vi "Subvi trigger AO DO.vi"(9 "Ext trig enable":bool) -> ()   [LabVIEW 2017]
uses:
  <vilib>/Platform/TimedLoop/XDataNode/timing_clust.ctl
  <vilib>/Platform/TimedLoop/XDataNode/nitl_modes.ctl
  <vilib>/Platform/TimedLoop/XDataNode/wakeup.ctl
  <vilib>/rvi/Emulation/niFpgaSctlEmulationGetInTimedLoop.vi
  <vilib>/rvi/Emulation/niFpgaEmulationReportErrorSimple.vi
  <vilib>/rvi/Emulation/niFpgaGetClockAttributes.vi
  <vilib>/rvi/Emulation/niFpgaCriticalErrorInLSC.vi
  Detector/GV preline gate.vi
  GV trigger delay.vi
  <vilib>/Platform/TimedLoop/XDataNode/XDataNode.xnode
  <vilib>/Platform/TimedLoop/XDataNode/XDNodeRunTimeDep.lvlib
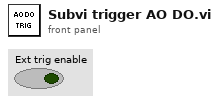
[diagram p1: front panel]
types:
  T1 = typedef "XDNodeRunTimeDep.lvlib/timing_clust.ctl" = cluster{"Expected End [f-1]":u64, "Actual End [f-1]":u64, "Finished Late? [f-1]":bool, "Expected End [i-1]":u64, "Actual End [i-1]":u64, "Finished Late? [i-1]":bool, "Expected Start [i]":u64, "Actual Start [i]":u64, "Expected Start [f]":u64, "Actual Start [f]":u64, "Source Name":string, "Structure Name":string, "Period":i64, "Deadline":i64, "Offset":i64, "Start":i64, "Priority":i32, "Timeout":i32, "Mode":T2, "Wakeup Reason":T3, "Error":errorcluster, "Source Type":string, "Secondary Source Type":string, "Global End Time":u64, "Global Start Time":u64, "Frame Duration":u64, "Iteration Duration":u64, "Assigned CPU":i32, "I/O Scan Engine Mode":u32}
  T2 = typedef "XDNodeRunTimeDep.lvlib/nitl_modes.ctl" = enum32{"No Change", "Process missed periods, maintain original phase", "Discard missed periods, maintain original phase", "Process missed periods, ignore original phase", "Discard missed periods, ignore original phase"}
  T3 = typedef "XDNodeRunTimeDep.lvlib/wakeup.ctl" = enum32{"Normal", "Aborted", "Asynchronous wakeup", "Timing source error", "Timed loop error", "Timeout"}
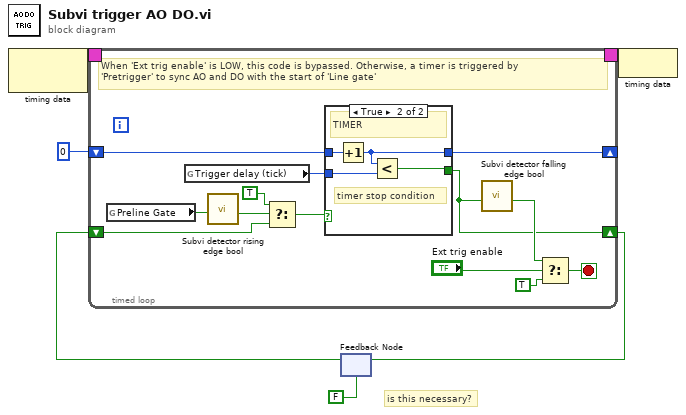
[diagram p0: block diagram]
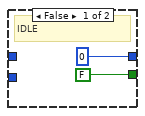
[diagram p2: hidden frame]
diagram:
  # "is this necessary?"
  n1 = node-c288() -> (w6:T1)  [unwired: 1 in]
  n2 = feedback #1(FALSE) -> (w2:bool)
  n3 = timed-loop {
    timing: w6 -> [_]
    timing-out: [_] -> w5
    shift-right: [w7] -> w1
    shift-left: w2 -> [w13]
    shift-right: [w16] -> _
    shift-left: u16 0 -> [w15]
    stop <- w11 stop-if-true
    # "When 'Ext trig enable' is LOW, this code is bypassed. Otherwise, a timer is triggered by\n'Pretrigger' to sync AO and DO with the start of 'Line gate'"
    n4 = global read "GV preline gate.vi" "Preline Gate"() -> (w8:bool)
    n5 = global read "GV trigger delay.vi" "Trigger delay (tick)"() -> (w14:u16)
    n6 = call "Subvi detector rising edge bool.vi"("Input"=w8) -> ("Output"=w17:bool)  [unwired: 10 in]
    n7 = Select(t=TRUE, s=w17, f=w13) -> (s? t:f=w18:bool)
    n8 = case shown="True" w18 {
      tunnel: [FALSE w23] -> w7
      tunnel: [u16 0 w24] -> w16
      tunnel: w15 -> [_ w25]
      tunnel: w14 -> [_ w22]
      frame False {
        # "IDLE"
      }
      frame True {
        # "timer stop condition"
        # "TIMER"
        n9 = Increment(x=w25) -> (x+1=w24:u16)
        n10 = Less?(x=w24, y=w22) -> (x < y?=w23:bool)
      }
    }
    n11 = call "Subvi detector falling edge bool.vi"("Input"=w7) -> ("Output"=w9:bool)  [unwired: 10 in]
    n12 = Select(t=w9, s="Ext trig enable", f=TRUE) -> (s? t:f=w11:bool)
  }
  n13 = feedback-in #1(w1) -> ()
  n14 = node-c288(w5) -> ()
